vi "Add Element.vi"(8 "error in":errorcluster, 10 "STEP":refnum<class "STEP.lvclass">, 11 "SEQ in":refnum<class "SEQ.lvclass">) -> (0 "error out":errorcluster, 3 "SEQ out":refnum<class "SEQ.lvclass">)   [LabVIEW 2015, in "Sequence Composition.lvlib" / "SEQ.lvclass"]
uses:
  SEQ.lvclass
  STEPS/STEP.lvclass
  STEPS/STEP.lvclass/STEP.ctl
  SEQ.lvclass/SEQ.ctl
  STEPS/Write First Call.vi
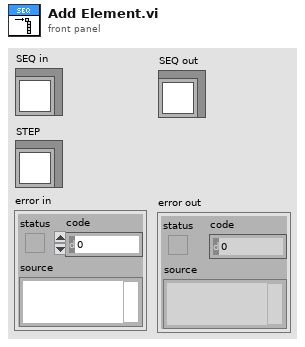
[diagram p1: front panel]
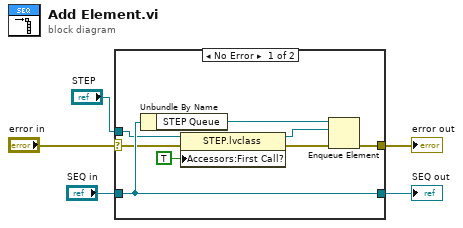
[diagram p0: block diagram]
diagram:
  n1 = case shown="No Error" "error in" {
    selector: "error in" -> [w9 w15]
    tunnel: [w11 w15] -> w4
    tunnel: [w13 w14] -> w2
    tunnel: "SEQ in" -> [w13 w14]
    tunnel: "STEP" -> [w10 _]
    frame No Error {
      n2 = Unbundle By Name(w13) -> ("STEP Queue"=w12:refnum<queue>)
      n3 = property class="STEP.lvclass"(reference=w10, error in=w9, "Accessors:First Call?"=TRUE ("First Call?")) -> (reference out=w8:refnum<class "STEP.lvclass">, error out=w7:errorcluster)
      n4 = Enqueue Element(queue=w12, element=w8, error in (no error)=w7) -> (error out=w11:errorcluster)  [unwired: 1 in, 2 out]
    }
    frame Error {
    }
  }
  "error out" <- w4
  "SEQ out" <- w2
